vi "Common.vi"(10 "xData in":refnum<class "xData.lvclass">, 11 "Controller in":refnum<class "Controller.lvclass">) -> ()   [LabVIEW 2018, in "Controller.lvlib" / "Controller.lvclass"]
doc: "This VI is intended to run all tasks common to the Controller. It should run parallel to the Actor Core.vi. While this VI is running, it will output a heartbeat that is visible via the Heartbeat LED."
uses:
  Controller.lvclass
  Update Controller Data MSG.lvclass
  <vilib>/ActorFramework/Message Enqueuer/Message Enqueuer.lvclass
  <vilib>/ActorFramework/Actor/Actor.lvclass
  reusable/Session APIs/Session Log/System Log.lvclass
  <vilib>/DAQmx/write.llb/DAQmx Write (Digital Bool 1Line 1Point).vi
  <vilib>/Analysis/NI_AALBase.lvlib
  <vilib>/Platform/TimedLoop/XDataNode/XDataNode.xnode
  <vilib>/Platform/TimedLoop/XDataNode/nitl_modes.ctl
  <vilib>/Platform/TimedLoop/XDataNode/XDNodeRunTimeDep.lvlib
  <vilib>/Platform/TimedLoop/XDataNode/wakeup.ctl
  <vilib>/Platform/TimedLoop/XDataNode/timing_clust.ctl
  Data/xData.lvclass
  <vilib>/DAQmx/read.llb/DAQmx Read (Digital 1D Bool NChan 1Samp 1Line).vi
  <vilib>/DAQmx/read.llb/DAQmx Read (Analog 1D DBL 1Chan NSamp).vi
  <vilib>/Analysis/baseanly.llb/Mean (DBL).vi
  <vilib>/Platform/TimedLoop/scheduler/LVUserAPI/_suppVIs/Create_1kHz_TSource.vi
  reusable/Session APIs/CVT/CVT.lvclass
  reusable/Session APIs/CVT/Get Boolean Array Data.vi
  reusable/Session APIs/CVT/Get Boolean Data.vi
  reusable/Switch/Switch.lvclass
  reusable/Session APIs/CVT/Get U8 Data.vi
  C:/Users/Labview/Documents/exscalabar_server/SuperActor/SuperActor.lvclass
  C:/Program Files (x86)/National Instruments/LabVIEW 2018/vi.lib/ActorFramework/Actor/Actor.lvclass
  C:/Users/Labview/Documents/exscalabar_server/reusable/Data/Data.lvclass
  C:/Users/Labview/Documents/exscalabar_server/reusable/DAQ Device/Device/Generic Data Update Data MSG/Generic Update Data Message.lvclass
  C:/Program Files (x86)/National Instruments/LabVIEW 2018/vi.lib/ActorFramework/Message/Message.lvclass
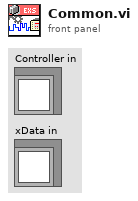
[diagram p1: front panel]
types:
  T1 = typedef "Session - Root.lvclass/Session Handle.ctl" = refnum<data-value>
  T2 = typedef "XDNodeRunTimeDep.lvlib/timing_clust.ctl" = cluster{"Expected End [f-1]":u64, "Actual End [f-1]":u64, "Finished Late? [f-1]":bool, "Expected End [i-1]":u64, "Actual End [i-1]":u64, "Finished Late? [i-1]":bool, "Expected Start [i]":u64, "Actual Start [i]":u64, "Expected Start [f]":u64, "Actual Start [f]":u64, "Source Name":string, "Structure Name":string, "Period":i64, "Deadline":i64, "Offset":i64, "Start":i64, "Priority":i32, "Timeout":i32, "Mode":T3, "Wakeup Reason":T4, "Error":errorcluster, "Source Type":string, "Secondary Source Type":string, "Global End Time":u64, "Global Start Time":u64, "Frame Duration":u64, "Iteration Duration":u64, "Assigned CPU":i32, "I/O Scan Engine Mode":u32}
  T3 = typedef "XDNodeRunTimeDep.lvlib/nitl_modes.ctl" = enum32{"No Change", "Process missed periods, maintain original phase", "Discard missed periods, maintain original phase", "Process missed periods, ignore original phase", "Discard missed periods, ignore original phase"}
  T4 = typedef "XDNodeRunTimeDep.lvlib/wakeup.ctl" = enum32{"Normal", "Aborted", "Asynchronous wakeup", "Timing source error", "Timed loop error", "Timeout"}
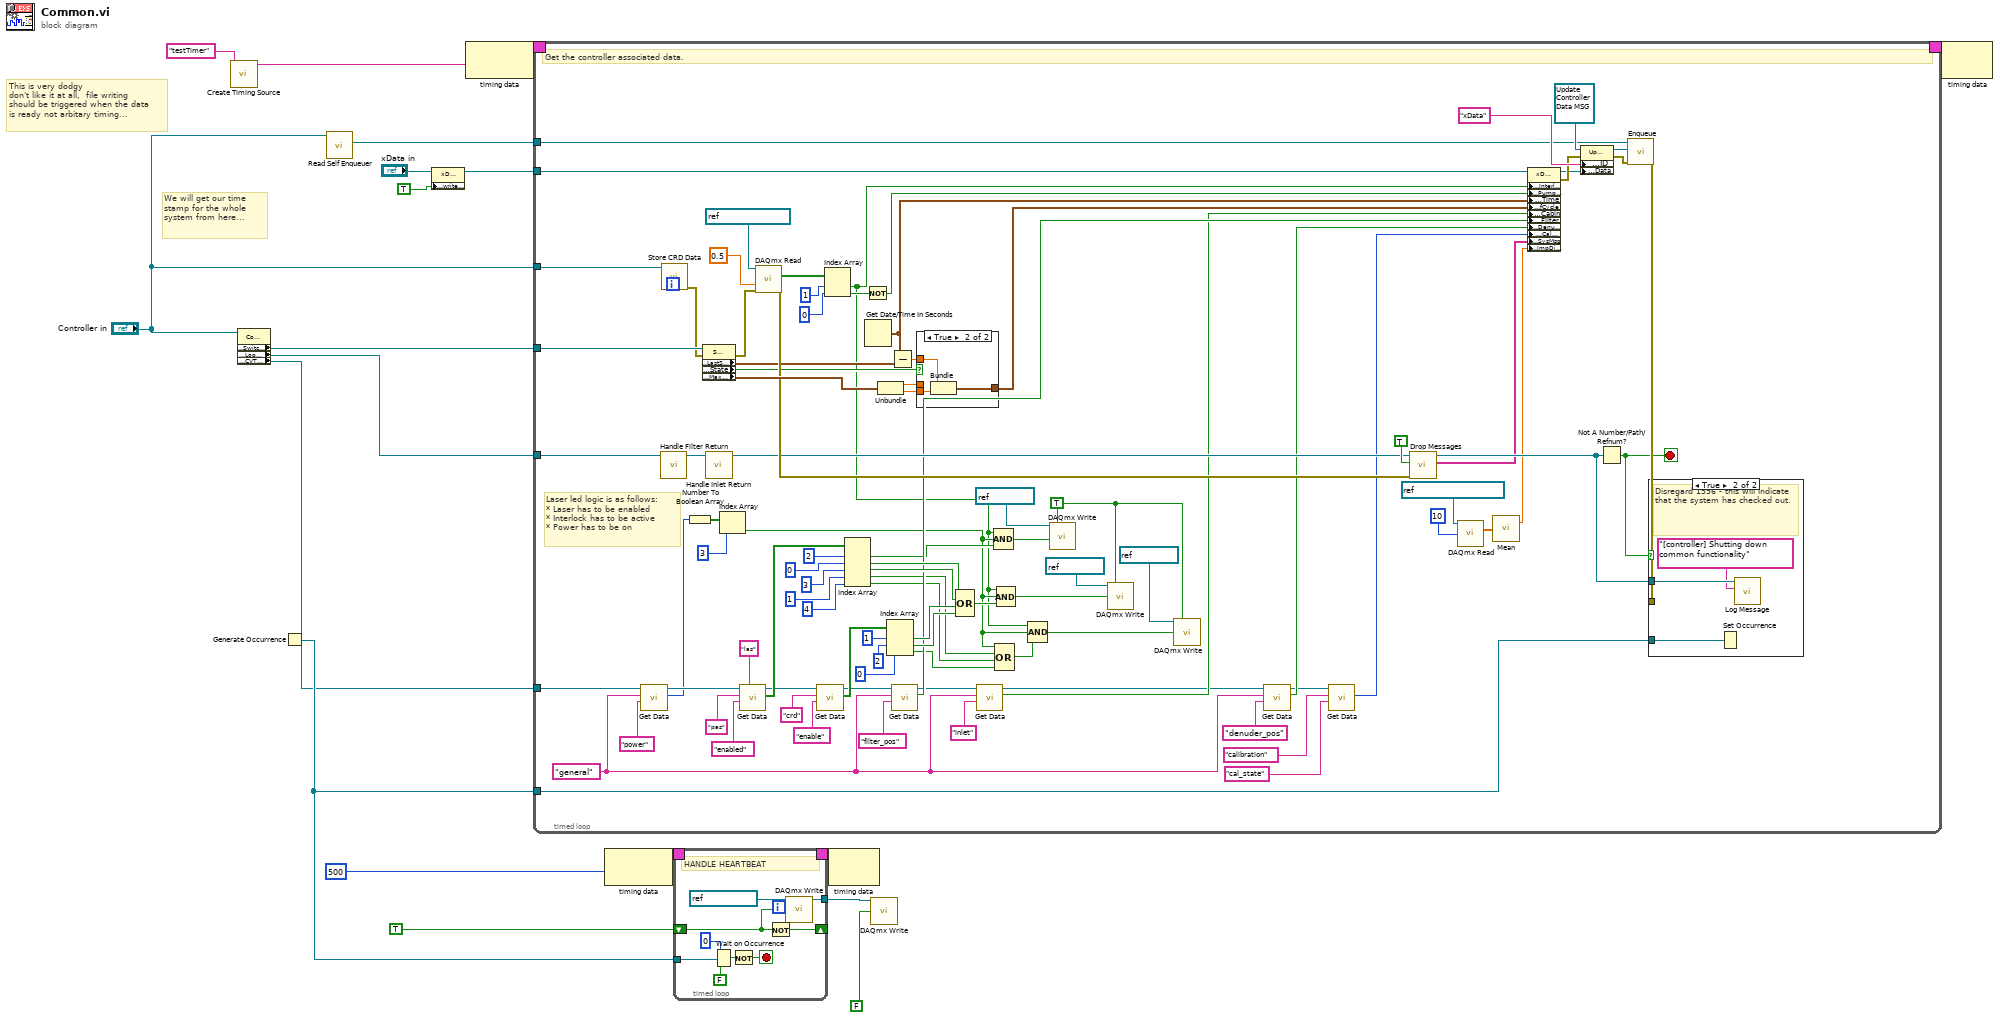
[diagram p0: block diagram]
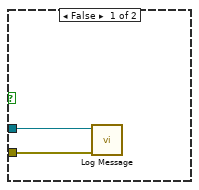
[diagram p2: hidden frame]
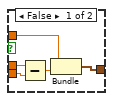
[diagram p3: hidden frame]
diagram:
  # "This is very dodgy \ndon't like it at all,  file writing\nshould be triggered when the data \nis ready not arbitary timing..."
  # "We will get our time stamp for the whole system from here..."
  n1 = call-poly <vilib>:"Create Timing Source.vi"("name (in)"="testTimer") -> ("name (out)"=w1:string)  [unwired: 9 in, 1 out]
  n2 = property class="Controller"(reference="Controller in") -> ("Accessors:Switch DVR"=w11:refnum<data-value>, "Accessors:Log Session"=w10:T1, "Accessors:CVT Session"=w3:T1)  [unwired: 1 in, 2 out]
  n3 = Generate Occurrence() -> (w12:refnum<k4>)
  n4 = call <vilib>:"Read Self Enqueuer.vi"("Actor"="Controller in") -> ("Self Enqueuer"=w19:refnum<class "Message Enqueuer.lvclass">)  [unwired: 10 in]
  n5 = property class="xData"(reference="xData in", "Accessors:write time"=TRUE ("write time")) -> (reference out=w6:refnum<class "xData.lvclass">)  [unwired: 1 in, 1 out]
  n6 = node-c288(w1) -> (w18:T2)
  n7 = timed-loop {
    tunnel: w6 -> [w105]
    tunnel: w19 -> [w82]
    tunnel: w10 -> [w85]
    tunnel: w11 -> [w103]
    tunnel: "Controller in" -> [w97]
    timing: w18 -> [_]
    timing-out: [_] -> w17
    tunnel: w12 -> [w87]
    tunnel: w3 -> [w34]
    stop <- w80 stop-if-true
    w32 = "general" ("Group")
    w37 = TRUE ("auto start")
    # "Laser led logic is as follows: \n* Laser has to be enabled\n* Interlock has to be active\n* Power has to be on"
    # "Get the controller associated data."
    n8 = call-poly "Get Data.vi"("Variable"="power", "Group"=w32, "CVT Session In"=w34) -> ("U8"=w30:u8, "CVT Session Out"=w33:T1)  [unwired: 5 in, 2 out]
    n9 = call "Handle Filter Return.vi"("Log Session"=w85) -> ("Log Session Out"=w84:T1)  [unwired: 8 in, 2 out]
    n10 = call "Store CRD Data.vi"("Controller in"=w97) -> ("error out"=w93:errorcluster)  [unwired: 9 in, 1 out]
    n11 = Number To Boolean Array(number=w30) -> (Boolean array=w29:bool[])
    n12 = property class="Switch"(reference=w103, error in=w93) -> (error out=w92:errorcluster, "Accessors:LastSwitch"=w88:timestamp, "Data Access:State"=w89:bool, "Data Access:Max Elapsed Time"=w102:cluster{"Period":sgl, "Length":sgl})  [unwired: 1 out]
    n13 = call "Handle Inlet Return.vi"("Log Session"=w84) -> ("Log Session Out"=w83:T1)  [unwired: 8 in, 2 out]
    n14 = Index Array(array=w29, index=3) -> (element=w22:bool)
    n15 = call-poly "Get Data.vi"("Subgroup"="las", "Variable"="enabled", "Group"="pas", "CVT Session In"=w33) -> ("Boolean Array"=w58:bool[], "CVT Session Out"=w57:T1)  [unwired: 4 in, 2 out]
    n16 = call-poly <vilib>:"DAQmx Read.vi"("task/channels in"=refnum<k21> "General Input", "timeout"=0.5, "error in"=w92) -> ("data"=w111:bool[], "error out"=w91:errorcluster)  [unwired: 10 in, 1 out]
    n17 = call-poly "Get Data.vi"("Variable"="enable", "Group"="crd", "CVT Session In"=w57) -> ("Boolean Array"=w54:bool[], "CVT Session Out"=w53:T1)  [unwired: 5 in, 2 out]
    n18 = Index Array(array=w111, index #1=1 ("index"), index #2=0 ("index")) -> (element #1=w21:bool, element #2=w86:bool)
    n19 = Index Array(array=w58, index #1=2 ("index"), index #2=0 ("index"), index #3=3 ("index"), index #4=1 ("index"), index #5=4 ("index")) -> (element #1=w26:bool, element #2=w74:bool, element #3=w73:bool, element #4=w38:bool, element #5=w40:bool)
    n20 = Not(x=w86) -> (.not. x?=w64:bool)
    n21 = Get Date/Time In Seconds() -> (seconds since 1Jan1904=w63:timestamp)
    n22 = Unbundle(w102) -> ("Period"=w99:sgl, "Length"=w100:sgl)
    n23 = Index Array(array=w54, index #1=1 ("index"), index #2=2 ("index"), index #3=0 ("index")) -> (element #1=w70:bool, element #2=w69:bool, element #3=w39:bool)
    n24 = Subtract(x=w63, y=w88) -> (x-y=w101:dbl)
    n25 = call-poly "Get Data.vi"("Variable"="filter_pos" ("tag"), "Group"=w32, "CVT Session In"=w53) -> ("Boolean"=w51:bool, "CVT Session Out"=w50:T1)  [unwired: 5 in, 2 out]
    n26 = case shown="True" w89 {
      tunnel: w101 -> [w125 w128]
      tunnel: w100 -> [w124 w127]
      tunnel: w99 -> [w123 _]
      tunnel: [w121 w126] -> w62
      frame False {
        n27 = Subtract(x=w123, y=w124) -> (x-y=w122:sgl)
        n28 = Bundle(w125, w122) -> (w121:cluster{dbl, sgl})  [unwired: 1 in]
      }
      frame True {
        n29 = Bundle(w128, "Length"=w127) -> (w126:cluster{dbl, "Length":sgl})  [unwired: 1 in]
      }
    }
    n30 = Compound Arithmetic op=OR(w74, w73, w70, w69) -> (w27:bool)
    n31 = call-poly "Get Data.vi"("Variable"="inlet" ("tag"), "Group"=w32, "CVT Session In"=w50) -> ("Boolean"=w48:bool, "CVT Session Out"=w47:T1)  [unwired: 5 in, 2 out]
    n32 = Compound Arithmetic op=AND(w21, w22, w26) -> (w25:bool)
    n33 = Compound Arithmetic op=OR(w22, w38, w40, w39) -> (w23:bool)
    n34 = Compound Arithmetic op=AND(w21, w22, w27) -> (w24:bool)
    n35 = Compound Arithmetic op=AND(w21, w22, w23) -> (w20:bool)
    n36 = call-poly <vilib>:"DAQmx Write.vi"("task/channels in"=refnum<k21> "515 LED", "auto start"=w37, "data"=w25) -> ()  [unwired: 10 in, 3 out]
    n37 = call-poly <vilib>:"DAQmx Write.vi"("task/channels in"=refnum<k21> "405 LED", "auto start"=w37, "data"=w24) -> ()  [unwired: 10 in, 3 out]
    n38 = call-poly <vilib>:"DAQmx Write.vi"("task/channels in"=refnum<k21> "660 LED", "auto start"=w37, "data"=w20) -> ()  [unwired: 10 in, 3 out]
    n39 = call-poly "Get Data.vi"("Variable"="denuder_pos" ("tag"), "Group"=w32, "CVT Session In"=w47) -> ("Boolean"=w45:bool, "CVT Session Out"=w44:T1)  [unwired: 5 in, 2 out]
    n40 = call-poly "Get Data.vi"("Variable"="cal_state" ("Group"), "Group"="calibration" ("Subgroup"), "CVT Session In"=w44) -> ("U8"=w41:u8)  [unwired: 5 in, 3 out]
    n41 = call "Drop Messages.vi"("error in"=w91, "Drop?"=TRUE, "log in"=w83) -> ("Current Msgs"=w36:string[], "log out"=w81:T1)  [unwired: 6 in, 1 out]
    n42 = call-poly <vilib>:"DAQmx Read.vi"("task/channels in"=refnum<k21> "Blocked Impactor", "number of samples per channel"=10) -> ("data"=w95:dbl[])  [unwired: 11 in, 2 out]
    n43 = call-poly <vilib>:"Mean.vi"("X"=w95) -> ("mean"=w35:dbl)  [unwired: 1 out]
    n44 = property class="xData"(reference=w105, "Accessors:Interlock"=w21, "Accessors:PumpBlocked"=w64, "Accessors:Time"=w63, "Accessors:fCycle"=w62, "Accessors:Cabin"=w48, "Accessors:Filter"=w51, "Accessors:DenuderBypass"=w45, "Accessors:Cal State"=w41, "Accessors:SysMsg"=w36, "Accessors:ImpDiffV"=w35) -> (reference out=w107:refnum<class "xData.lvclass">, error out=w108:errorcluster)  [unwired: 1 in]
    n45 = property class="Update Data MSG"(reference=refnum<class "Update Controller Data MSG.lvclass"> refnum ("Controller.lvlib:Update Data MSG"), error in=w108, "Accessors:ID"="xData" ("ID"), "Accessors:Data"=w107) -> (reference out=w106:refnum<class "Update Controller Data MSG.lvclass">, error out=w98:errorcluster)
    n46 = Not A Number/Path/Refnum?(number/path/refnum=w81) -> (NaN/Path/Refnum?=w80:bool)
    n47 = call <vilib>:"Enqueue.vi"("error in (no error)"=w98, "Message"=w106, "Message Enqueuer in"=w82) -> ("error out"=w90:errorcluster)  [unwired: 7 in, 1 out]
    n48 = case shown="True" w80 {
      tunnel: w81 -> [w117 w120]
      tunnel: w90 -> [w116 _]
      tunnel: w87 -> [_ w118]
      frame False {
        n49 = call "Log Message.vi"("error in"=w116, "session in"=w117) -> ()  [unwired: 8 in, 2 out]
      }
      frame True {
        # "Disregard 1556 - this will indicate that the system has checked out."
        n50 = Set Occurrence(w118) -> ()
        n51 = call "Log Message.vi"("MSG In"="[controller] Shutting down common functionality", "session in"=w120) -> ()  [unwired: 8 in, 2 out]
      }
    }
  }
  n52 = node-c288(i64 500 ("Period")) -> (w15:T2)
  n53 = timed-loop {
    shift-right: [w138] -> _
    shift-left: TRUE -> [w139]
    timing: w15 -> [_]
    timing-out: [_] -> w14
    tunnel: w12 -> [w136]
    tunnel: [w131] -> w9
    stop <- w133 stop-if-true
    # "HANDLE HEARTBEAT"
    n54 = Wait on Occurrence(1:FALSE ("ignore previous (T)"), 2:w136, 3:0 ("ms timeout (-1)")) -> (0:w134:bool)
    n55 = Not(x=w134) -> (.not. x?=w133:bool)
    n56 = Not(x=w139) -> (.not. x?=w138:bool)
    n57 = call-poly <vilib>:"DAQmx Write.vi"("task/channels in"=refnum<k21> "Heartbeat", "data"=w139) -> ("task out"=w131:refnum<k21>)  [unwired: 11 in, 2 out]
  }
  n58 = node-c288(w14) -> ()  [unwired: 1 out]
  n59 = call-poly <vilib>:"DAQmx Write.vi"("task/channels in"=w9, "data"=FALSE) -> ()  [unwired: 11 in, 3 out]
  n60 = node-c288(w17) -> ()  [unwired: 1 out]
